vi "Generate Event.vi"(4 "Error In":errorcluster) -> (0 "Error Out":errorcluster)   [LabVIEW 2015, in "ude_Handle Errors.lvlib"]
uses:
  ude_Handle Errors.lvlib
  Event Data.ctl
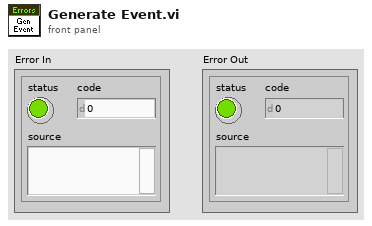
[diagram p1: front panel]
types:
  T1 = typedef "ude_Handle Errors.lvlib/Event Data.ctl" = cluster{"Error Data":errorcluster}
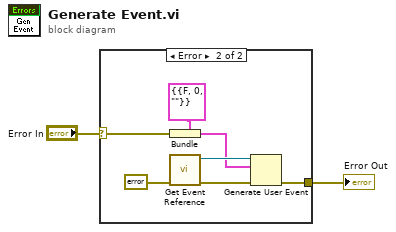
[diagram p0: block diagram]
diagram:
  n1 = case shown="Error" "Error In" {
    selector: "Error In" -> [w3 w6]
    tunnel: [w3 w8] -> w2
    frame No Error {
    }
    frame Error {
      n2 = Bundle(cluster=T1 {"Error Data"={"status"=FALSE, "code"=0, "source"=""}} ("event data"), "Error Data"=w6) -> (w4:T1)
      n3 = call "Get Event Reference.vi"("error in (no error)"=errorcluster {"status"=FALSE, "code"=0, "source"=""}) -> ("error out"=w10:errorcluster, "System Error"=w9:refnum<user-event>)  [unwired: 5 in]
      n4 = Generate User Event(user event=w9, event data cluster=w4, error in=w10) -> (error out=w8:errorcluster)  [unwired: 1 in, 1 out]
    }
  }
  "Error Out" <- w2
